vi "AngleBetweenFits.vi"(8 "Slope 2":dbl, 11 "Slope 1":dbl) -> ()   [LabVIEW 2016]
panel:
  out "arcseconds":dbl
  out "arcminutes":dbl
  out "Degrees":dbl
  out "Angle (Degrees)":dbl
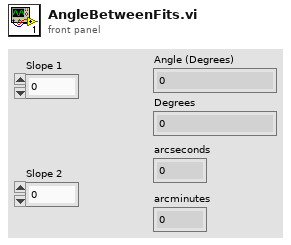
[diagram p1: front panel]
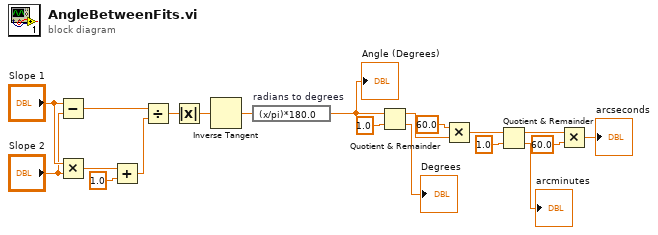
[diagram p0: block diagram]
diagram:
  n1 = Subtract(x="Slope 1", y="Slope 2") -> (x-y=w16:dbl)
  n2 = Multiply(x="Slope 1", y="Slope 2") -> (x*y=w18:dbl)
  n3 = Add(x=w18, y=1.0) -> (x+y=w15:dbl)
  n4 = Divide(x=w16, y=w15) -> (x/y=w14:dbl)
  n5 = Absolute Value(x=w14) -> (abs(x)=w13:dbl)
  n6 = Inverse Tangent(1:w13) -> (0:w10:dbl)
  n7 = expression code="(x/pi)*180.0" "radians to degrees"(w10) -> (w9:dbl)
  "Angle (Degrees)" <- w9
  n8 = Quotient & Remainder(x=w9, y=1.0) -> (x-y*floor(x/y)=w7:dbl, floor(x/y)=→"Degrees":dbl)
  n9 = Multiply(x=60.0 ("y"), y=w7) -> (x*y=w6:dbl)
  n10 = Quotient & Remainder(x=w6, y=1.0) -> (x-y*floor(x/y)=w2:dbl, floor(x/y)=→"arcminutes":dbl)
  n11 = Multiply(x=w2, y=60.0) -> (x*y=→"arcseconds":dbl)
